vi "Main.vi"() -> ()   [LabVIEW 2021]
uses:
  TypeDefs/DevInfo.ctl
  TypeDefs/TargetAccess.ctl
  <vilib>/nisyscfg/Network Settings Format.ctl
  f3a6a675-c2de-4d38-9339-871dcd676738.vi
  <userlib>/S2 Labs/Error Reporting/Transport_WinDebug/Transport_WinDebug.lvclass
  C:/Program Files (x86)/National Instruments/LabVIEW 2021/user.lib/S2 Labs/Error Reporting/Transport Class/Transport.lvclass
  <vilib>/nisyscfg/Close (System).vi
  <vilib>/nisyscfg/Format 5.3.vi
  <vilib>/nisyscfg/Save Changes (Hardware).vi
  <vilib>/nisyscfg/Close (Hardware).vi
  <vilib>/nisyscfg/Save Changes (System).vi
  <resource>/objmgr/nisysapi.rc
  <vilib>/nisyscfg/nisyscfg.lvlib
  <userlib>/S2 Labs/Error Reporting/Error Reporting.lvlib
  <resource>/objmgr/nicontrollersysapi.rc
panel:
  out "Refreshing":bool
  in  "Device List":i32(listbox)
  in  "ChangeMode":bool
  out "MAC":string
  out "OS":string
  out "Firmware":string
  out "Status":string
  out "Version":string
  out "Description":string
  out "Title":string
  out "Model":string
  in  "ChangePassword":bool
  in  "ChangeMode":bool
  in  "Restart":bool
  in  "FormatDisk":bool
  in  "ManageFeeds":bool
  in  "DeplyFW":bool
  in  "NetworkSettings":bool
  in  "Refresh":bool
  in  "DeplyImg":bool
  in  "RetrieveImg":bool
  # "Device Properties"
  # "Image Properties"
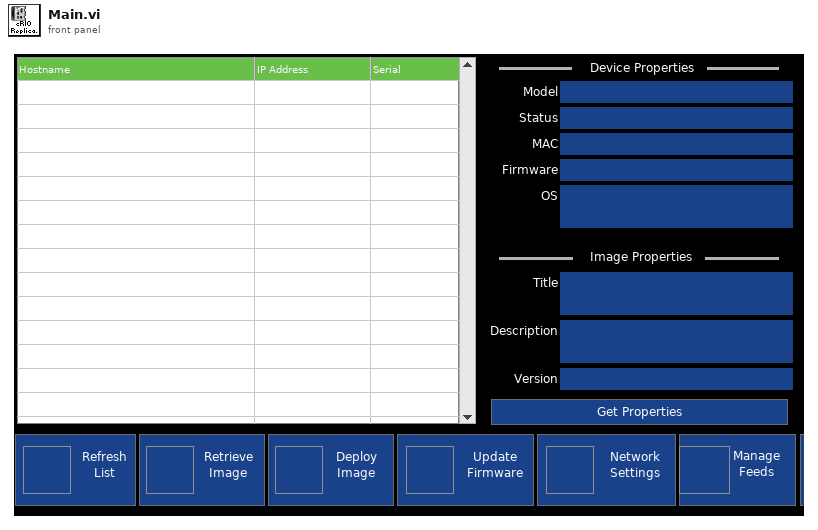
[diagram p1: front panel]
types:
  T1 = typedef "DevInfo.ctl" = cluster{"Hostname":string, "IPAddress":string, "MAC":string, "SerialNum":string, "Model":string, "Status":string, "FW":string, "OSDesc":string, "ImgTitle":string, "ImgDesc":string, "ImgVer":string, "ImgID":string, "IP Address Request Mode":i32, "SubnetMask":string, "Gateway":string, "DNSServer":string}
  T2 = enum8{"Enabled", "Disabled", "Disabled and Grayed Out"}
  T3 = typedef "TargetAccess.ctl" = enum16{"Read-Only", "Admin"}
  T4 = typedef "nisyscfg.lvlib/Network Settings Format.ctl" = u32
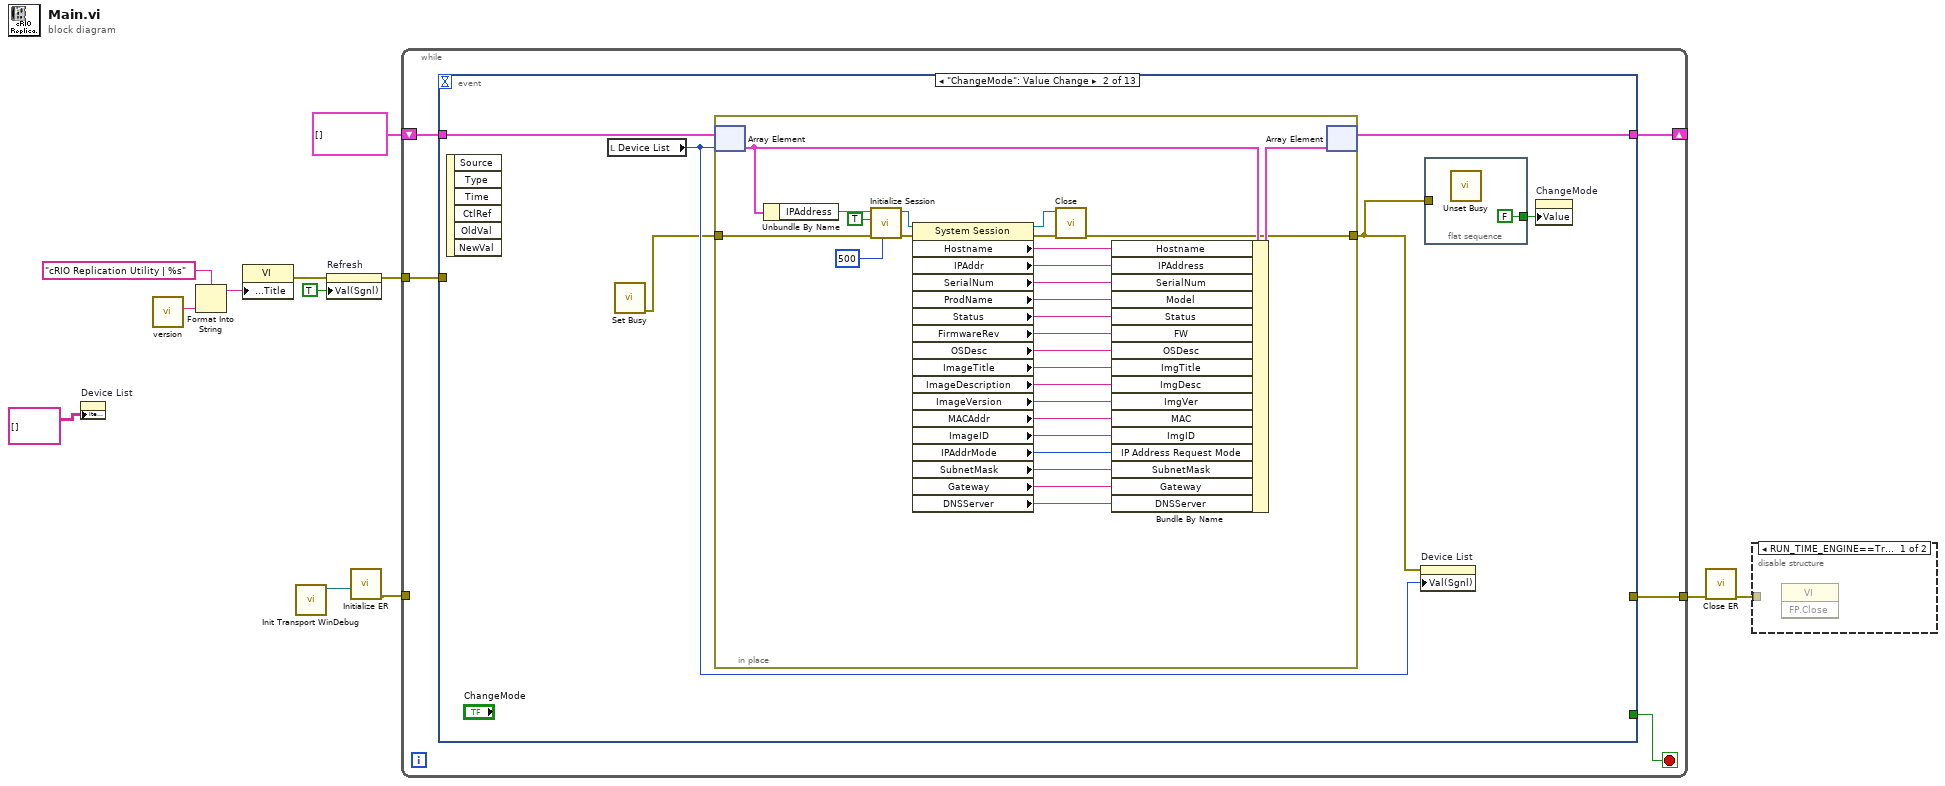
[diagram p0: block diagram]
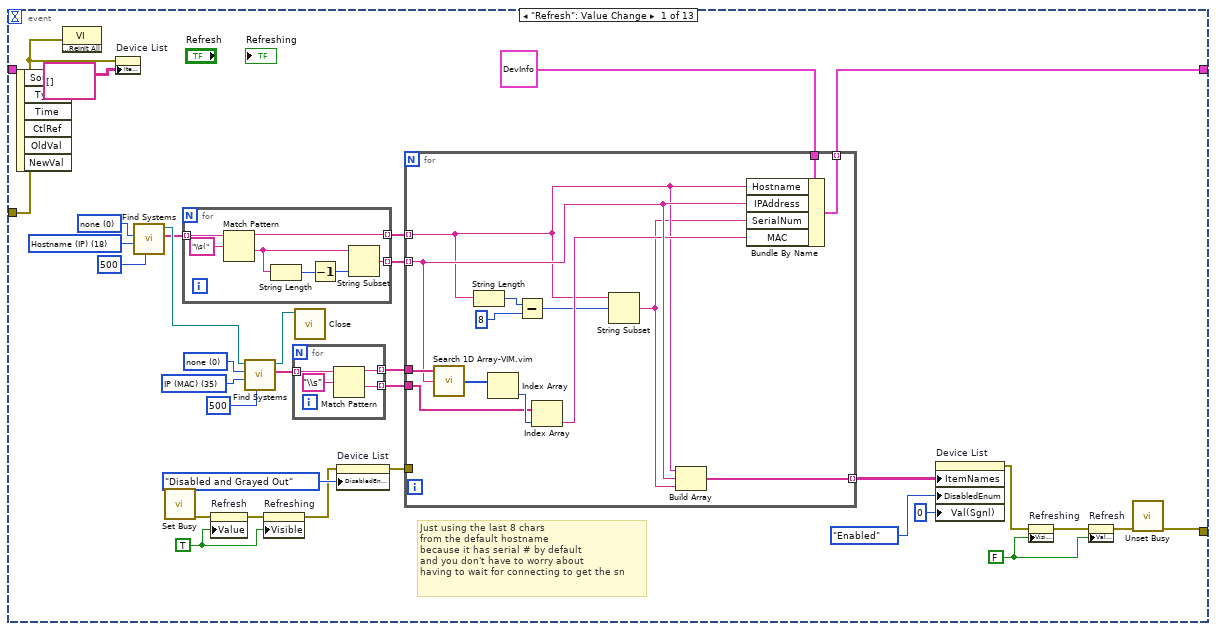
[diagram p3: hidden frame]
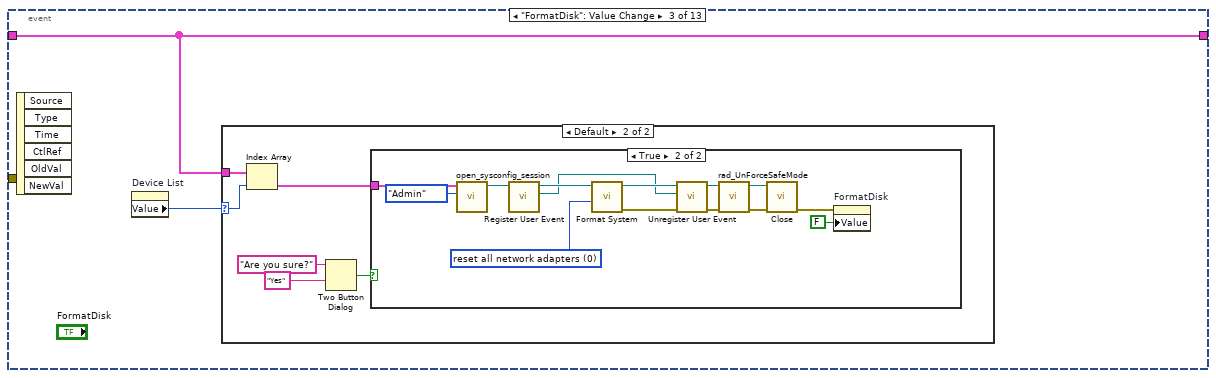
[diagram p4: hidden frame]
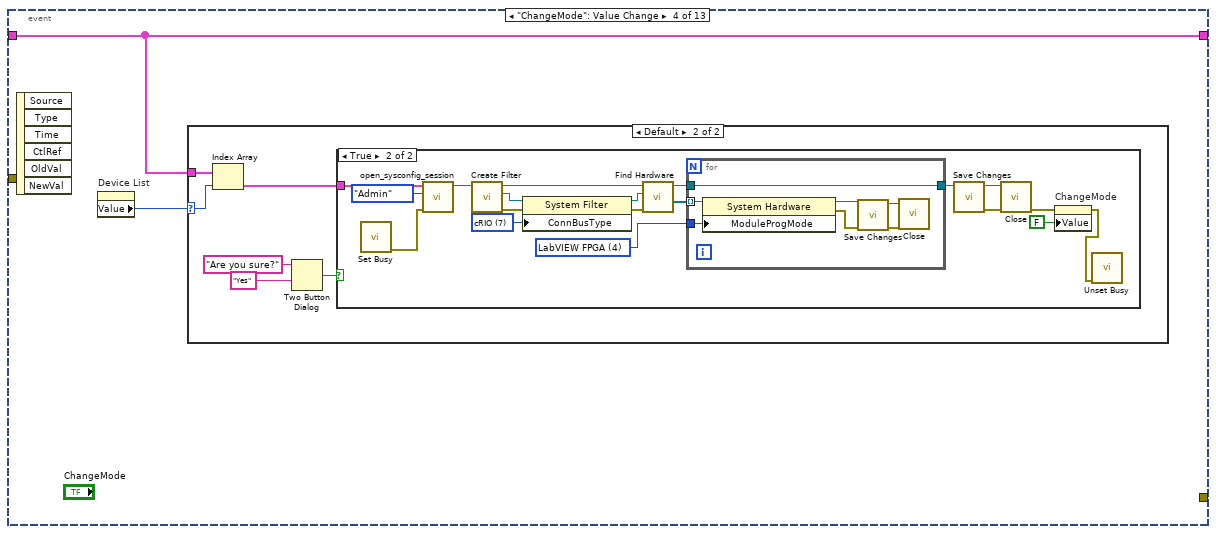
[diagram p7: hidden frame]
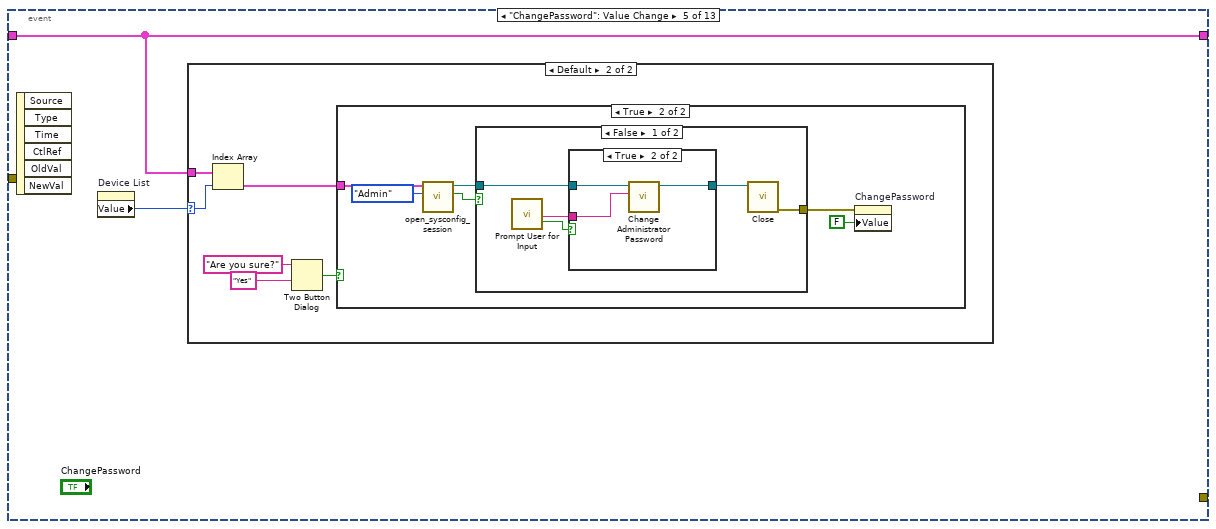
[diagram p10: hidden frame]
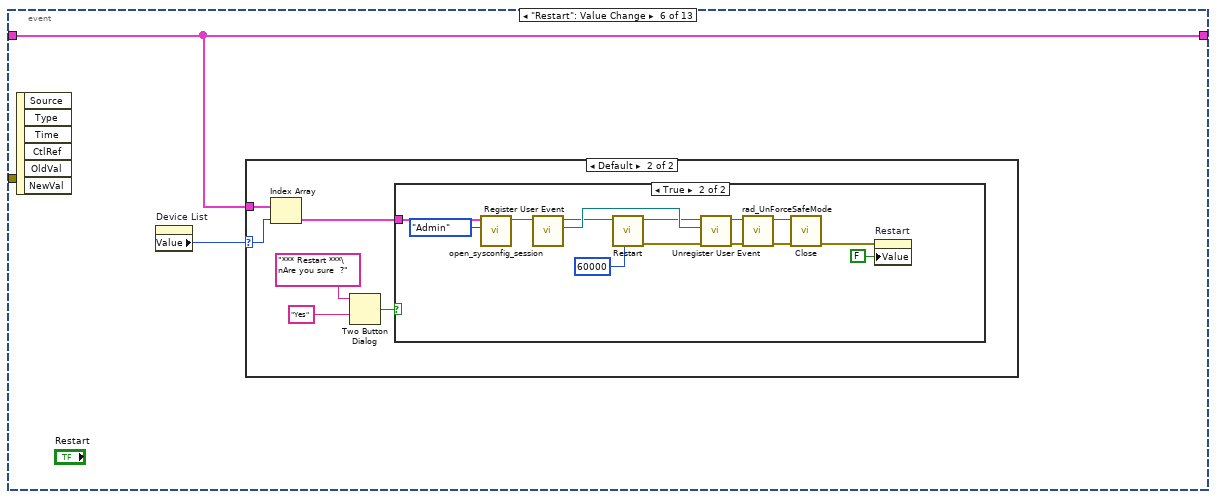
[diagram p15: hidden frame]
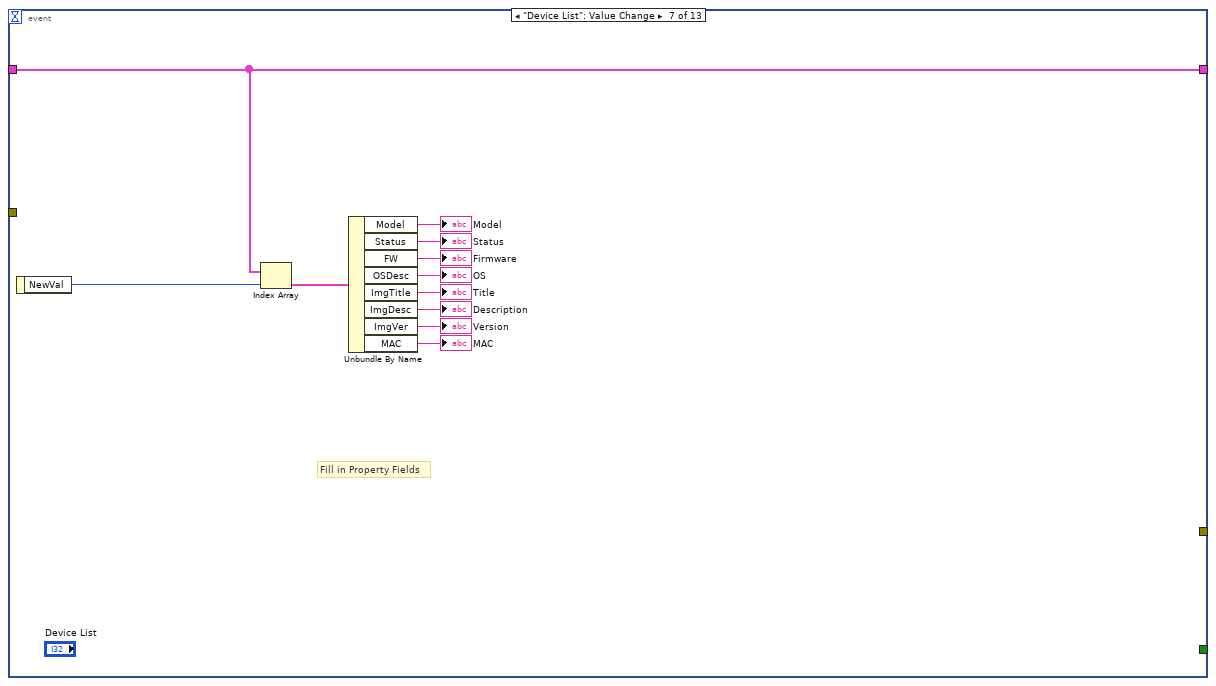
[diagram p18: hidden frame]
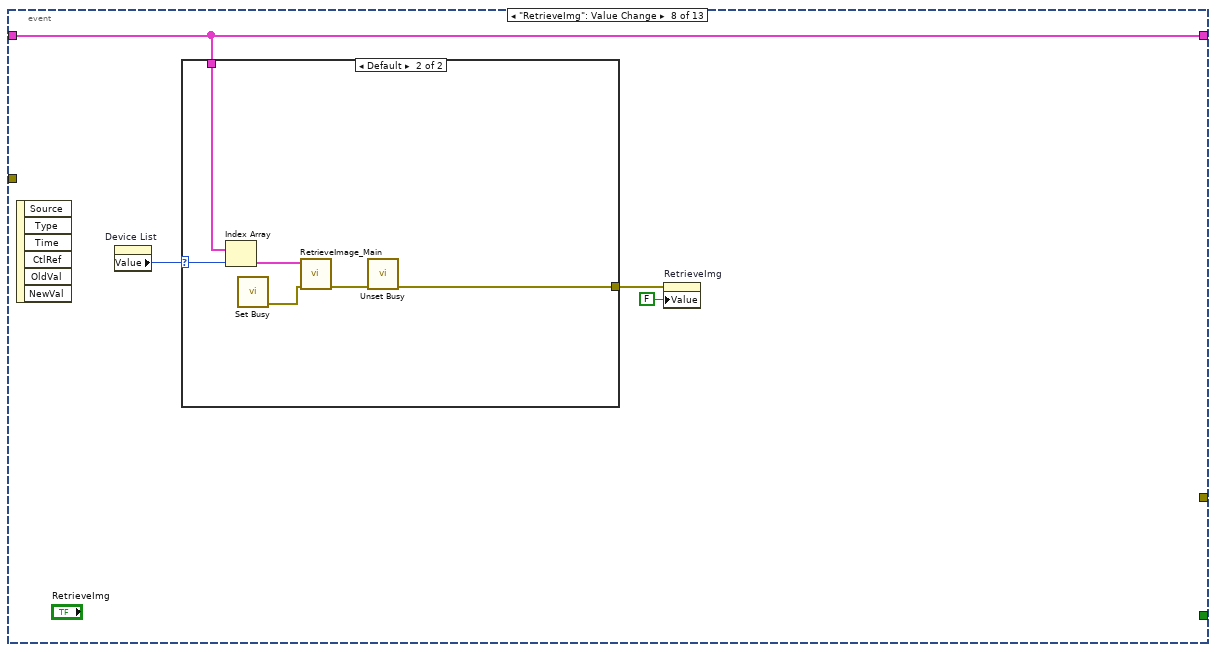
[diagram p19: hidden frame]
diagram:
  n1 = property on="Device List" class="MCListbox (strict)"("ItemNames"=string[][] [] ("Item Names")) -> ()  [unwired: 2 in, 2 out]
  n2 = call "version.vi"() -> ("version"=w6:string)  [unwired: 11 in]
  n3 = Format Into String(format string="cRIO Replication Utility | %s", w6) -> (resulting string=w5:string)  [unwired: 2 in, 1 out]
  n4 = property class="VI"("Front Panel.Title"=w5) -> (error out=w4:errorcluster)  [unwired: 2 in, 1 out]
  n5 = call <userlib>:"Init Transport WinDebug.vi"() -> ("Transport WinDebug"=w9:refnum<class "Transport_WinDebug.lvclass">)  [unwired: 11 in]
  n6 = property on="Refresh" class="Bool (strict)"(error in=w4, "Val(Sgnl)"=TRUE ("Value (Signaling)")) -> (error out=w3:errorcluster)  [unwired: 1 in, 1 out]
  n7 = call <userlib>:"Initialize ER.vi"("Transport Class (UDP)"=w9) -> ("error out"=w10:errorcluster)  [unwired: 10 in]
  n8 = while {
    shift-right: [w15] -> _
    shift-left: T1[] [] -> [w16]
    tunnel: w10 -> [_]
    tunnel: [w14] -> w8
    tunnel: w3 -> [w13]
    stop <- w17 stop-if-true
    n9 = event shown="[1] \"ChangeMode\": Value Change" {
      selector: _ -> [_ _ _ _ _ _ _ _ _ _ _ _ _]
      dyn-events: _ -> [_ _ _ _ _ _ _ _ _ _ _ _ _]
      timeout: _ -> [_ _ _ _ _ _ _ _ _ _ _ _ _]
      tunnel: [_ _ _ _ _ _ _ _ _ _ _ _ TRUE] -> w17
      tunnel: w16 -> [_ w79 w109 w131 w165 w188 w220 w223 w233 w243 w253 w263 w272]
      tunnel: [w35 w80 w109 w131 w165 w188 w220 w223 w233 w243 w253 w263 w272] -> w15
      tunnel: [w33 _ _ _ _ _ _ _ _ _ _ _ errorcluster {"status"=FALSE, "code"=0, "source"=""} ("error out")] -> w14
      tunnel: w13 -> [w32 _ _ _ _ _ _ _ _ _ _ _ _]
      event "Refresh": Value Change {
        w25 = u32 0 items=["none"=0, "only if online"=1, "all"=3] ("Include Cached Results (all)")
        w26 = u32 35 items=["Hostname"=16, "Hostname (IP)"=18, "Hostname (MAC)"=19, "IP"=32, "IP (Hostname)"=33, "IP (MAC)"=35, "MAC"=48, "MAC (Hostname)"=49, "MAC (IP)"=50] ("Output (Hostname and IP)")
        w22 = u32 0 items=["none"=0, "only if online"=1, "all"=3] ("Include Cached Results (all)")
        w23 = u32 18 items=["Hostname"=16, "Hostname (IP)"=18, "Hostname (MAC)"=19, "IP"=32, "IP (Hostname)"=33, "IP (MAC)"=35, "MAC"=48, "MAC (Hostname)"=49, "MAC (IP)"=50] ("Output (Hostname and IP)")
        w41 = FALSE ("Visible")
        w42 = TRUE ("Visible")
        # "Just using the last 8 chars\nfrom the default hostname \nbecause it has serial # by default\nand you don't have to worry about\nhaving to wait for connecting to get the sn"
        n10 = event-data() -> ()  [unwired: 1 in, 6 out]
        n11 = invoke class="VI" method="Default Vals.Reinit All"(error in=w32) -> ()  [unwired: 2 in, 3 out]
        n12 = property on="Device List" class="MCListbox (strict)"(error in=w32, "ItemNames"=string[][] [] ("Item Names")) -> ()  [unwired: 1 in, 2 out]
        n13 = call <vilib>:"Find Systems.vi"("Timeout (4000 ms)"=u32 500, "Output (Hostname and IP)"=w23, "Include Cached Results (all)"=w22) -> ("Detected Systems"=w29:string[], "Session out"=w30:refnum<k21>)  [unwired: 6 in, 1 out]
        n14 = call <vilib>:"Set Busy.vi"() -> ("error out"=w39:errorcluster)  [unwired: 10 in, 1 out]
        n15 = for {
          tunnel: w29 -> [w60] mode=indexing
          tunnel: [w58] -> w21 mode=indexing
          tunnel: [w56] -> w20 mode=indexing
          n16 = Match Pattern(string=w60, regular expression="\\s(") -> (before substring=w58:string, after substring=w57:string)  [unwired: 1 in, 2 out]
          n17 = String Length(string=w57) -> (length=w55:i32)
          n18 = Decrement(x=w55) -> (x-1=w54:i32)
          n19 = String Subset(string=w57, length (rest)=w54) -> (substring=w56:string)  [unwired: 1 in]
        }
        n20 = property on="Refresh" class="Bool (strict)"(error in=w39, "Value"=w42) -> (error out=w43:errorcluster)  [unwired: 1 in, 1 out]
        n21 = call <vilib>:"Find Systems.vi"("Timeout (4000 ms)"=u32 500, "Output (Hostname and IP)"=w26, "Include Cached Results (all)"=w25, "Session in (localhost)"=w30) -> ("Detected Systems"=w28:string[], "Session out"=w31:refnum<k21>)  [unwired: 5 in, 1 out]
        n22 = property on="Refreshing" class="Bool (strict)"(error in=w43, "Visible"=w42) -> (error out=w45:errorcluster)  [unwired: 1 in, 1 out]
        n23 = for {
          tunnel: w28 -> [w52] mode=indexing
          tunnel: [w51] -> w19 mode=indexing
          tunnel: [w50] -> w18 mode=indexing
          n24 = Match Pattern(string=w52, regular expression="\\s") -> (before substring=w51:string, after substring=w50:string)  [unwired: 1 in, 2 out]
        }
        n25 = call-poly <vilib>:"Close.vi"("Session in"=w31) -> ()  [unwired: 10 in, 1 out]
        n26 = property on="Device List" class="MCListbox (strict)"(error in=w45, "DisabledEnum"=T2."Disabled and Grayed Out" ("Disabled")) -> (error out=w47:errorcluster)  [unwired: 1 in, 1 out]
        n27 = for {
          tunnel: [w74] -> w49 mode=indexing
          tunnel: w47 -> [_]
          tunnel: T1 {"Hostname"="", "IPAddress"="", "MAC"="", "SerialNum"="", "Model"="", "Status"="", "FW"="", "OSDesc"="", "ImgTitle"="", "ImgDesc"="", "ImgVer"="", "ImgID"="", "IP Address Request Mode"=1, "SubnetMask"="", "Gateway"="", "DNSServer"=""} ("DevInfo") -> [w73]
          tunnel: [w72] -> w35 mode=indexing
          tunnel: w21 -> [w63] mode=indexing
          tunnel: w20 -> [w67] mode=indexing
          tunnel: w19 -> [w68]
          tunnel: w18 -> [w69]
          n28 = call "Search 1D Array-VIM.vim"("Array"=w68, "Element Data"=w67) -> ("Indices of Elements"=w70:i32[])  [unwired: 7 in]
          n29 = String Length(string=w63) -> (length=w65:i32)
          n30 = Index Array(array=w70) -> (element=w71:i32)  [unwired: 1 in]
          n31 = Subtract(x=w65, y=8) -> (x-y=w62:i32)
          n32 = Index Array(array=w69, index=w71) -> (element=w66:string)
          n33 = String Subset(string=w63, offset (0)=w62) -> (substring=w61:string)  [unwired: 1 in]
          n34 = Build Array(w63, w67, w61) -> (w74:string[])
          n35 = Bundle By Name(cluster=w73, "Hostname"=w63, "IPAddress"=w67, "SerialNum"=w61, "MAC"=w66) -> (w72:T1)
        }
        n36 = property on="Device List" class="MCListbox (strict)"("ItemNames"=w49, "DisabledEnum"=T2."Enabled" ("Disabled"), "Val(Sgnl)"=0 ("Value (Signaling)")) -> (error out=w44:errorcluster)  [unwired: 2 in, 1 out]
        n37 = property on="Refreshing" class="Bool (strict)"(error in=w44, "Visible"=w41) -> (error out=w40:errorcluster)  [unwired: 1 in, 1 out]
        n38 = property on="Refresh" class="Bool (strict)"(error in=w40, "Value"=w41) -> (error out=w38:errorcluster)  [unwired: 1 in, 1 out]
        n39 = call <vilib>:"Unset Busy.vi"("error in (no error)"=w38) -> ("error out"=w33:errorcluster)  [unwired: 10 in]
      }
      event "ChangeMode": Value Change {
        n40 = event-data() -> ()  [unwired: 1 in, 6 out]
        n41 = local read "Device List"() -> (w78:i32)
        n42 = call <vilib>:"Set Busy.vi"() -> ("error out"=w77:errorcluster)  [unwired: 10 in, 1 out]
        n43 = in-place {
          in-place-border: [w83] -> w76
          in-place-border: w77 -> [w82]
          n44 = in-place-array #1(w79, w78) -> (w85:T1)
          n45 = Unbundle By Name(w85) -> ("IPAddress"=w94:string)
          n46 = call <vilib>:"Initialize Session.vi"("Connect Timeout (4000 ms)"=u32 500, "error in (no error)"=w82, "Force Property Refresh (T)"=TRUE, "Target (localhost)"=w94) -> ("error out"=w105:errorcluster, "Session out"=w108:refnum<k21>)  [unwired: 6 in]
          n47 = property class="System Session"(reference=w108, error in=w105) -> (reference out=w107:refnum<k21>, error out=w104:errorcluster, "Hostname"=w102:string, "IPAddr"=w101:string, "SerialNum"=w100:string, "ProdName"=w95:string, "Status"=w99:string, "FirmwareRev"=w98:string, "OSDesc"=w97:string, "ImageTitle"=w96:string, "ImageDescription"=w93:string, "ImageVersion"=w92:string, "MACAddr"=w91:string, "ImageID"=w90:string, "IPAddrMode"=w89:i32, "SubnetMask"=w88:string, "Gateway"=w87:string, "DNSServer"=w86:string)
          n48 = call-poly <vilib>:"Close.vi"("error in (no error)"=w104, "Session in"=w107) -> ("error out"=w83:errorcluster)  [unwired: 9 in]
          n49 = Bundle By Name(cluster=w85, "Hostname"=w102, "IPAddress"=w101, "SerialNum"=w100, "Model"=w95, "Status"=w99, "FW"=w98, "OSDesc"=w97, "ImgTitle"=w96, "ImgDesc"=w93, "ImgVer"=w92, "MAC"=w91, "ImgID"=w90, "IP Address Request Mode"=w89, "SubnetMask"=w88, "Gateway"=w87, "DNSServer"=w86) -> (w84:T1)
          n50 = in-place-array #1(w84) -> (w80:T1[])  [unwired: 1 out]
        }
        n51 = property on="Device List" class="MCListbox (strict)"(error in=w76, "Val(Sgnl)"=w78) -> ()  [unwired: 1 in, 2 out]
        n52 = flat-sequence {
          tunnel: w76 -> [_]
          tunnel: [FALSE ("ChangeMode")] -> w75
          frame #0 {
            n53 = call <vilib>:"Unset Busy.vi"() -> ()  [unwired: 11 in, 1 out]
          }
        }
        n54 = property on="ChangeMode" class="Bool (strict)"("Value"=w75) -> ()  [unwired: 2 in, 2 out]
      }
      event "FormatDisk": Value Change {
        n55 = event-data() -> ()  [unwired: 1 in, 6 out]
        n56 = property on="Device List" class="MCListbox (strict)"() -> ("Value"=w110:i32)  [unwired: 2 in, 2 out]
        n57 = case shown="Default" w110 {
          selector: w110 -> [_ w115]
          tunnel: w109 -> [_ w116]
          frame -1 {
          }
          frame Default {
            n58 = Index Array(array=w116, index=w115) -> (element=w111:T1)
            n59 = Two Button Dialog(message="Are you sure?", 2:"Yes" ("T button name (\"OK\")")) -> (T button?=w112:bool)  [unwired: 1 in]
            n60 = case shown="True" w112 {
              tunnel: w111 -> [_ w128]
              frame False {
              }
              frame True {
                w127 = T4 0 items=["reset all network adapters", "preserve primary, reset others", "preserve all network adapters"] ("Network Settings (reset all adapters)")
                n61 = call "open_sysconfig_session.vi"("Target Access"=TargetAccess."Admin", "DevInfo"=w128) -> ("Session Out"=w129:refnum<k21>)  [unwired: 7 in, 2 out]
                n62 = call <vilib>:"Register User Event.vi"("Session in"=w129) -> ("Event Registration out"=w119:refnum<event-registration>, "Session out"=w126:refnum<k21>)  [unwired: 8 in, 1 out]
                n63 = call-poly <vilib>:"Format System.vi"("Network Settings (reset all adapters)"=w127, "Session in"=w126) -> ("error out"=w123:errorcluster, "Session out"=w122:refnum<k21>)  [unwired: 8 in]
                n64 = call <vilib>:"Unregister User Event.vi"("error in (no error)"=w123, "Event Registration in"=w119, "Session in"=w122) -> ("error out"=w124:errorcluster, "Session out"=w125:refnum<k21>)  [unwired: 7 in]
                n65 = call "rad_UnForceSafeMode.vi"("error in (no error)"=w124, "Target in"=w125) -> ("error out"=w120:errorcluster, "Target out"=w121:refnum<k21>)  [unwired: 8 in]
                n66 = call-poly <vilib>:"Close.vi"("error in (no error)"=w120, "Session in"=w121) -> ("error out"=w118:errorcluster)  [unwired: 9 in]
                n67 = property on="FormatDisk" class="Bool (strict)"(error in=w118, "Value"=FALSE ("FormatDisk")) -> ()  [unwired: 1 in, 2 out]
              }
            }
          }
        }
      }
      event "ChangeMode": Value Change {
        n68 = event-data() -> ()  [unwired: 1 in, 6 out]
        n69 = property on="Device List" class="MCListbox (strict)"() -> ("Value"=w132:i32)  [unwired: 2 in, 2 out]
        n70 = case shown="Default" w132 {
          selector: w132 -> [_ w137]
          tunnel: w131 -> [_ w138]
          frame -1 {
          }
          frame Default {
            n71 = Index Array(array=w138, index=w137) -> (element=w133:T1)
            n72 = Two Button Dialog(message="Are you sure?", 2:"Yes" ("T button name (\"OK\")")) -> (T button?=w134:bool)  [unwired: 1 in]
            n73 = case shown="True" w134 {
              tunnel: w133 -> [_ w156]
              frame False {
              }
              frame True {
                w144 = u32 4 items=["None"=0, "Real-Time CPU"=1, "Real-Time Scan Engine"=2, "LabVIEW FPGA"=4] ("Devices & Chassis:Bus Specific:cRIO Module Programming Mode")
                w143 = u32 7 items=["BuiltIn/System", "PXI/PCI", "USB", "GPIB", "VXI", "Serial", "TCP/IP", "cRIO", "SCXI", "cDAQ", "SwitchBlock", "SCC", "FireWire", "Accessory", "CAN", "SwitchBlock Device", "SLSC"] ("Devices & Chassis:Connects To Bus Type")
                n74 = call <vilib>:"Set Busy.vi"() -> ("error out"=w140:errorcluster)  [unwired: 10 in, 1 out]
                n75 = call "open_sysconfig_session.vi"("error in (no error)"=w140, "Target Access"=TargetAccess."Admin", "DevInfo"=w156) -> ("Session Out"=w142:refnum<k21>)  [unwired: 6 in, 2 out]
                n76 = call <vilib>:"Create Filter.vi"("Session in"=w142) -> ("error out"=w145:errorcluster, "Filter out"=w146:refnum<k20>, "Session out"=w149:refnum<k21>)  [unwired: 8 in]
                n77 = property class="System Filter"(reference=w146, error in=w145, "ConnBusType"=w143) -> (reference out=w148:refnum<k20>, error out=w147:errorcluster)
                n78 = call <vilib>:"Find Hardware.vi"("error in (no error)"=w147, "Filter in"=w148, "Session in"=w149) -> ("Resources out"=w150:refnum<k20>[], "Session out"=w151:refnum<k21>)  [unwired: 5 in, 2 out]
                n79 = for {
                  tunnel: w150 -> [w164] mode=indexing
                  tunnel: w151 -> [w159]
                  tunnel: [w159] -> w152
                  tunnel: w144 -> [w158]
                  n80 = property class="System Hardware"(reference=w164, "ModuleProgMode"=w158) -> (reference out=w161:refnum<k20>, error out=w163:errorcluster)  [unwired: 1 in]
                  n81 = call-poly <vilib>:"Save Changes.vi"("error in (no error)"=w163, "Resource in"=w161) -> ("error out"=w160:errorcluster, "Resource out"=w162:refnum<k20>)  [unwired: 6 in, 2 out]
                  n82 = call-poly <vilib>:"Close.vi"("error in (no error)"=w160, "Resource in"=w162) -> ()  [unwired: 9 in, 1 out]
                }
                n83 = call-poly <vilib>:"Save Changes.vi"("Session in"=w152) -> ("error out"=w154:errorcluster, "Session out"=w153:refnum<k21>)  [unwired: 7 in, 2 out]
                n84 = call-poly <vilib>:"Close.vi"("error in (no error)"=w154, "Session in"=w153) -> ("error out"=w141:errorcluster)  [unwired: 9 in]
                n85 = property on="ChangeMode" class="Bool (strict)"(error in=w141, "Value"=FALSE ("FormatDisk")) -> (error out=w139:errorcluster)  [unwired: 1 in, 1 out]
                n86 = call <vilib>:"Unset Busy.vi"("error in (no error)"=w139) -> ()  [unwired: 10 in, 1 out]
              }
            }
          }
        }
      }
      event "ChangePassword": Value Change {
        n87 = event-data() -> ()  [unwired: 1 in, 6 out]
        n88 = property on="Device List" class="MCListbox (strict)"() -> ("Value"=w166:i32)  [unwired: 2 in, 2 out]
        n89 = case shown="Default" w166 {
          selector: w166 -> [_ w171]
          tunnel: w165 -> [_ w172]
          frame -1 {
          }
          frame Default {
            n90 = Index Array(array=w172, index=w171) -> (element=w167:T1)
            n91 = Two Button Dialog(message="Are you sure?", 2:"Yes" ("T button name (\"OK\")")) -> (T button?=w168:bool)  [unwired: 1 in]
            n92 = case shown="True" w168 {
              tunnel: w167 -> [_ w177]
              frame False {
              }
              frame True {
                n93 = call "open_sysconfig_session.vi"("Target Access"=TargetAccess."Admin", "DevInfo"=w177) -> ("Cancelled"=w173:bool, "Session Out"=w174:refnum<k21>)  [unwired: 7 in, 1 out]
                n94 = case shown="False" w173 {
                  tunnel: [w183 _] -> w175
                  tunnel: w174 -> [w182 _]
                  frame False {
                    n95 = call "Prompt User for Input"() -> ("New Password"=w180:string, "OK"=w179:bool)  [unwired: 17 in, 1 out]
                    n96 = case shown="True" w179 {
                      tunnel: w182 -> [w184 w187]
                      tunnel: [w184 w186] -> w181
                      tunnel: w180 -> [_ w185]
                      frame False {
                      }
                      frame True {
                        n97 = call <vilib>:"Change Administrator Password.vi"("New Password"=w185, "Session in"=w187) -> ("Session out"=w186:refnum<k21>)  [unwired: 8 in, 1 out]
                      }
                    }
                    n98 = call-poly <vilib>:"Close.vi"("Session in"=w181) -> ("error out"=w183:errorcluster)  [unwired: 10 in]
                  }
                  frame True {
                  }
                }
                n99 = property on="ChangePassword" class="Bool (strict)"(error in=w175, "Value"=FALSE ("FormatDisk")) -> ()  [unwired: 1 in, 2 out]
              }
            }
          }
        }
      }
      event "Restart": Value Change {
        n100 = event-data() -> ()  [unwired: 1 in, 6 out]
        n101 = property on="Device List" class="MCListbox (strict)"() -> ("Value"=w189:i32)  [unwired: 2 in, 2 out]
        n102 = case shown="Default" w189 {
          selector: w189 -> [_ w194]
          tunnel: w188 -> [_ w195]
          frame -1 {
          }
          frame Default {
            n103 = Index Array(array=w195, index=w194) -> (element=w190:T1)
            n104 = Two Button Dialog(message="*** Restart ***\nAre you sure  ?", 2:"Yes" ("T button name (\"OK\")")) -> (T button?=w191:bool)  [unwired: 1 in]
            n105 = case shown="True" w191 {
              tunnel: w190 -> [_ w207]
              frame False {
              }
              frame True {
                n106 = call "open_sysconfig_session.vi"("Target Access"=TargetAccess."Admin", "DevInfo"=w207) -> ("Session Out"=w208:refnum<k21>)  [unwired: 7 in, 2 out]
                n107 = call <vilib>:"Register User Event.vi"("Session in"=w208) -> ("Event Registration out"=w202:refnum<event-registration>, "Session out"=w201:refnum<k21>)  [unwired: 8 in, 1 out]
                n108 = call <vilib>:"Restart.vi"("Timeout (180,000 ms)"=u32 60000, "Session in"=w201) -> ("error out"=w199:errorcluster, "Session out"=w200:refnum<k21>)  [unwired: 7 in, 1 out]
                n109 = call <vilib>:"Unregister User Event.vi"("error in (no error)"=w199, "Event Registration in"=w202, "Session in"=w200) -> ("error out"=w205:errorcluster, "Session out"=w206:refnum<k21>)  [unwired: 7 in]
                n110 = call "rad_UnForceSafeMode.vi"("error in (no error)"=w205, "Target in"=w206) -> ("error out"=w203:errorcluster, "Target out"=w204:refnum<k21>)  [unwired: 8 in]
                n111 = call-poly <vilib>:"Close.vi"("error in (no error)"=w203, "Session in"=w204) -> ("error out"=w196:errorcluster)  [unwired: 9 in]
                n112 = property on="Restart" class="Bool (strict)"(error in=w196, "Value"=FALSE ("Restart")) -> ()  [unwired: 1 in, 2 out]
              }
            }
          }
        }
      }
      event "Device List": Value Change {
        # "Fill in Property Fields"
        n113 = event-data() -> ("NewVal"=w219:i32)  [unwired: 1 in]
        n114 = Index Array(array=w220, index=w219) -> (element=w218:T1)
        n115 = Unbundle By Name(w218) -> ("Model"=→"Model":string, "Status"=→"Status":string, "FW"=→"Firmware":string, "OSDesc"=→"OS":string, "ImgTitle"=→"Title":string, "ImgDesc"=→"Description":string, "ImgVer"=→"Version":string, "MAC"=→"MAC":string)
      }
      event "RetrieveImg": Value Change {
        n116 = event-data() -> ()  [unwired: 1 in, 6 out]
        n117 = property on="Device List" class="MCListbox (strict)"() -> ("Value"=w224:i32)  [unwired: 2 in, 2 out]
        n118 = case shown="Default" w224 {
          selector: w224 -> [_ w229]
          tunnel: w223 -> [_ w230]
          tunnel: [_ w225] -> w221
          frame -1 {
          }
          frame Default {
            n119 = Index Array(array=w230, index=w229) -> (element=w228:T1)
            n120 = call <vilib>:"Set Busy.vi"() -> ("error out"=w227:errorcluster)  [unwired: 10 in, 1 out]
            n121 = call "RetrieveImage_Main.vi"("error in (no error)"=w227, "DevInfo"=w228) -> ("error out"=w226:errorcluster)  [unwired: 9 in]
            n122 = call <vilib>:"Unset Busy.vi"("error in (no error)"=w226) -> ("error out"=w225:errorcluster)  [unwired: 10 in]
          }
        }
        n123 = property on="RetrieveImg" class="Bool (strict)"(error in=w221, "Value"=FALSE ("RetrieveImg")) -> ()  [unwired: 1 in, 2 out]
      }
      event "DeplyImg": Value Change {
        n124 = event-data() -> ()  [unwired: 1 in, 6 out]
        n125 = property on="Device List" class="MCListbox (strict)"() -> ("Value"=w234:i32)  [unwired: 2 in, 2 out]
        n126 = case shown="Default" w234 {
          selector: w234 -> [_ w239]
          tunnel: w233 -> [_ w240]
          tunnel: [_ w235] -> w231
          frame -1 {
          }
          frame Default {
            n127 = Index Array(array=w240, index=w239) -> (element=w238:T1)
            n128 = call <vilib>:"Set Busy.vi"() -> ("error out"=w237:errorcluster)  [unwired: 10 in, 1 out]
            n129 = call "DeployImage_Main.vi"("error in (no error)"=w237, "DevInfo"=w238) -> ("error out"=w236:errorcluster)  [unwired: 9 in]
            n130 = call <vilib>:"Unset Busy.vi"("error in (no error)"=w236) -> ("error out"=w235:errorcluster)  [unwired: 10 in]
          }
        }
        n131 = property on="DeplyImg" class="Bool (strict)"(error in=w231, "Value"=FALSE ("DeplyImg")) -> ()  [unwired: 1 in, 2 out]
      }
      event "DeplyFW": Value Change {
        n132 = event-data() -> ()  [unwired: 1 in, 6 out]
        n133 = property on="Device List" class="MCListbox (strict)"() -> ("Value"=w244:i32)  [unwired: 2 in, 2 out]
        n134 = case shown="Default" w244 {
          selector: w244 -> [_ w249]
          tunnel: w243 -> [_ w250]
          tunnel: [_ w248] -> w241
          frame -1 {
          }
          frame Default {
            n135 = Index Array(array=w250, index=w249) -> (element=w245:T1)
            n136 = call <vilib>:"Set Busy.vi"() -> ("error out"=w247:errorcluster)  [unwired: 10 in, 1 out]
            n137 = call "UpgradeFirmware_Main.vi"("error in (no error)"=w247, "DevInfo"=w245) -> ("error out"=w246:errorcluster)  [unwired: 9 in]
            n138 = call <vilib>:"Unset Busy.vi"("error in (no error)"=w246) -> ("error out"=w248:errorcluster)  [unwired: 10 in]
          }
        }
        n139 = property on="DeplyFW" class="Bool (strict)"(error in=w241, "Value"=FALSE ("DeplyImg")) -> ()  [unwired: 1 in, 2 out]
      }
      event "ManageFeeds": Value Change {
        n140 = event-data() -> ()  [unwired: 1 in, 6 out]
        n141 = property on="Device List" class="MCListbox (strict)"() -> ("Value"=w254:i32)  [unwired: 2 in, 2 out]
        n142 = case shown="Default" w254 {
          selector: w254 -> [_ w257]
          tunnel: w253 -> [_ w258]
          tunnel: [_ w255] -> w251
          frame -1 {
          }
          frame Default {
            n143 = Index Array(array=w258, index=w257) -> (element=w256:T1)
            n144 = call "Feed_Main.vi"("DevInfo"=w256) -> ("error out"=w255:errorcluster)  [unwired: 10 in]
          }
        }
        n145 = property on="ManageFeeds" class="Bool (strict)"(error in=w251, "Value"=FALSE ("ManageFeeds")) -> ()  [unwired: 1 in, 2 out]
      }
      event "NetworkSettings": Value Change {
        n146 = event-data() -> ()  [unwired: 1 in, 6 out]
        n147 = property on="Device List" class="MCListbox (strict)"() -> ("Value"=w264:i32)  [unwired: 2 in, 2 out]
        n148 = case shown="Default" w264 {
          selector: w264 -> [_ w269]
          tunnel: w263 -> [_ w270]
          tunnel: [_ w267] -> w259
          tunnel: [_ w266] -> w262
          frame -1 {
          }
          frame Default {
            n149 = Index Array(array=w270, index=w269) -> (element=w268:T1)
            n150 = call "Network_Main.vi"("DevInfo"=w268) -> ("error out"=w267:errorcluster, "Cancelled"=w266:bool)  [unwired: 9 in]
          }
        }
        n151 = Or(x=w262, y=w259) -> (x .or. y?=w260:bool)
        n152 = property on="NetworkSettings" class="Bool (strict)"(error in=w259, "Value"=FALSE ("DeplyImg")) -> ()  [unwired: 1 in, 2 out]
        n153 = case shown="False" w260 {
          frame False {
            n154 = property on="Refresh" class="Bool (strict)"("Val(Sgnl)"=TRUE ("Value (Signaling)")) -> ()  [unwired: 2 in, 2 out]
          }
          frame True {
          }
        }
      }
      event Panel Close? {
        n155 = event-data() -> ()  [unwired: 1 in, 4 out]
        n156 = event-data("Discard?"=TRUE) -> ()  [unwired: 1 in, 1 out]
      }
    }
  }
  n157 = call <userlib>:"Close ER.vi"("error in (no error)"=w8) -> ("error out"=w2:errorcluster)  [unwired: 10 in]
  n158 = disable-structure shown="RUN_TIME_ENGINE==True" {
    disable-tunnel: w2 -> [_ _]
    frame condition #0 {
      n159 = invoke class="VI" method="FP.Close"() -> ()  [unwired: 3 in, 3 out]
    }
    frame condition #1 (active) {
    }
  }
